vi "Test OOP API.vi"() -> ()   [LabVIEW 2019, in "Panther Dashboard.lvlib"]
uses:
  Panther Dashboard.lvlib
  <vilib>/National Instruments/Tree Map/API/List Roots.vi
  <vilib>/National Instruments/Tree Map/Utility/Into Tree Control Items.vi
  Class/VI/VI.lvclass
  Class/Library/Library.lvclass
  Class/Project/Project.lvclass
  <vilib>/National Instruments/Tree Map/Tree Map.lvlib
panel:
  in  "Modules Tree":string(tree)
  in  "error in":errorcluster
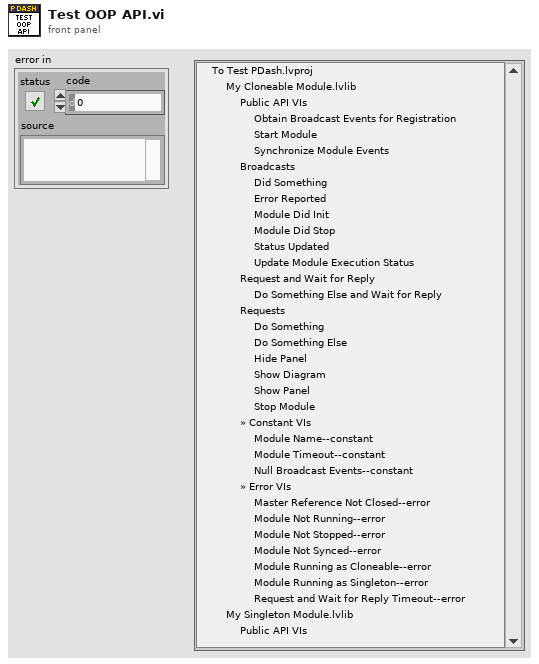
[diagram p1: front panel]
types:
  T1 = typedef "DQMH_Scripting API.lvlib/Module Information--cluster.ctl" = cluster{"Library":refnum<vi>, "Qualified Name":string, "Path":path, "Cloneable":bool, "Under Dependencies":bool}
  T2 = typedef "Tree Map.lvlib/Tree Map Data.ctl" = map{string, cluster{"Child Paths Set":set{string}, "Name":string, "Data":string, "Attributes":map{string, string}}}
  T3 = cluster{"Left Cell String":string, "Child Text":string[], "Child Tag":string, "Item Indent":i32, "Child Only?":bool, "Glyph Index":i32}[]
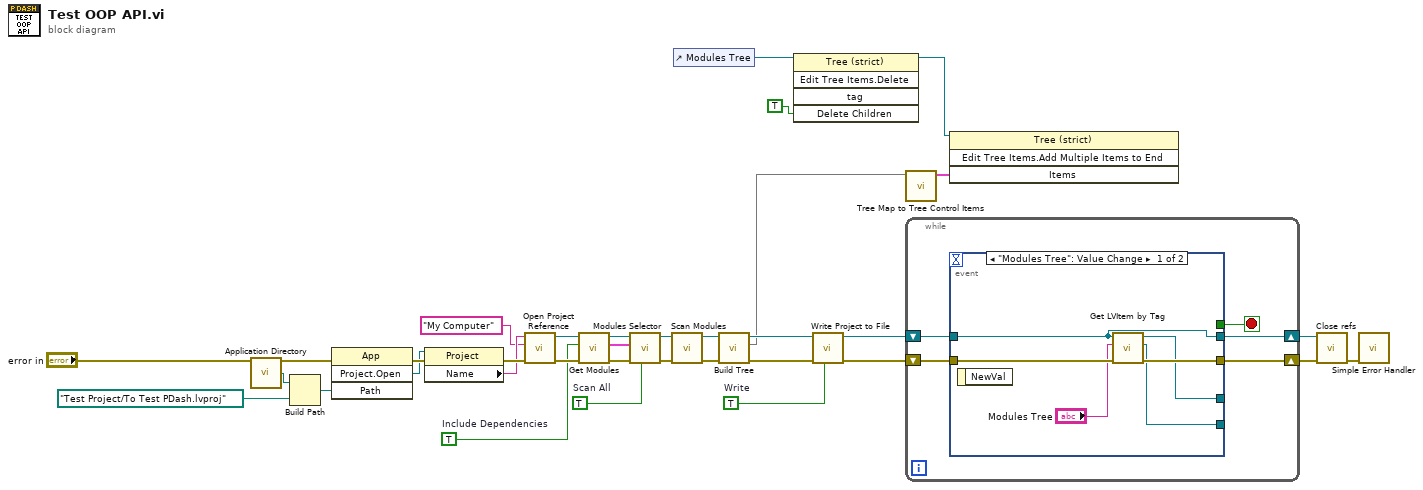
[diagram p0: block diagram]
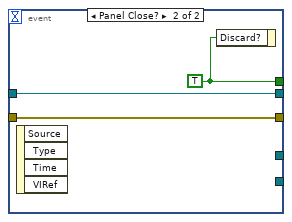
[diagram p2: hidden frame]
diagram:
  w2 = TRUE  # Write
  w19 = TRUE  # Scan All
  w17 = TRUE  # Include Dependencies
  n1 = call <vilib>:"Application Directory.vi"() -> ("Application Directory"=w16:path)
  n2 = Build Path(base path=w16, name or relative path=path "Test Project/To Test PDash.lvproj") -> (appended path=w14:path)
  n3 = invoke class="App" method="Project.Open"(error in="error in", "Path"=w14) -> (error out=w32:errorcluster, "Project:Open"=w13:refnum<vi>)  [unwired: 2 in, 2 out]
  n4 = property class="Project"(reference=w13, error in=w32) -> (error out=w30:errorcluster, "Name"=w12:string)  [unwired: 1 out]
  n5 = call "Open Project Reference.vi"("error in"=w30, "Target Selection"="My Computer", "Project Selection"=w12) -> ("error out"=w33:errorcluster, "Project"=w22:refnum<class "Project.lvclass">)  [unwired: 7 in]
  n6 = call "Get Modules.vi"("error in"=w33, "Include Dependencies"=w17, "Project in"=w22) -> ("error out"=w28:errorcluster, "DQMH Modules"=w20:T1[], "Project out"=w21:refnum<class "Project.lvclass">)  [unwired: 6 in]
  n7 = call "Modules Selector.vi"("Scan All"=w19, "error in"=w28, "DQMH Modules"=w20, "Project In"=w21) -> ("error out"=w27:errorcluster, "Project Out"=w18:refnum<class "Project.lvclass">)  [unwired: 5 in, 1 out]
  n8 = call "Scan Modules.vi"("error in (no error)"=w27, "Project In"=w18) -> ("error out"=w26:errorcluster, "Project Out"=w10:refnum<class "Project.lvclass">)  [unwired: 8 in]
  n9 = control-ref of="Modules Tree"() -> (w8:refnum<vi>)
  n10 = call "Build Tree.vi"("error in"=w26, "Project in"=w10) -> ("error out"=w24:errorcluster, "Tree Map Out"=w1:T2, "Project Out"=w4:refnum<class "Project.lvclass">)  [unwired: 7 in]
  n11 = invoke class="Tree (strict)" method="Edit Tree Items.Delete"(reference=w8, "Delete Children"=TRUE ("Delete Children?")) -> (reference out=w7:refnum<vi>)  [unwired: 3 in, 4 out]
  n12 = call "Write Project to File.vi"("Write"=w2, "error in"=w24, "Project In"=w4) -> ("error out"=w23:errorcluster, "Project Out"=w3:refnum<class "Project.lvclass">)  [unwired: 6 in, 1 out]
  n13 = call <vilib>:"Tree Map to Tree Control Items.vi"("Tree Map In"=w1) -> ("Tree Control Items"=w9:T3)  [unwired: 10 in]
  n14 = while {
    shift-right: [w37] -> w25
    shift-left: w23 -> [w38]
    shift-right: [w34] -> w5
    shift-left: w3 -> [w35]
    stop <- w36 stop-if-true
    n15 = event shown="[0] \"Modules Tree\": Value Change" {
      selector: _ -> [_ _]
      dyn-events: _ -> [_ _]
      timeout: _ -> [_ _]
      tunnel: w38 -> [w44 w47]
      tunnel: [w43 w47] -> w37
      tunnel: [_ w46] -> w36
      tunnel: w35 -> [w40 w45]
      tunnel: [w40 w45] -> w34
      tunnel: [w41 _] -> _
      tunnel: [w39 _] -> _
      event "Modules Tree": Value Change {
        n16 = event-data() -> ()  [unwired: 1 in, 1 out]
        n17 = call "Get LVItem by Tag.vi"("error in"=w44, "Tag"="Modules Tree", "Project in"=w40) -> ("error out"=w43:errorcluster, "Selected Library"=w41:refnum<class "Library.lvclass">, "Selected VI"=w39:refnum<class "VI.lvclass">)  [unwired: 6 in]
      }
      event Panel Close? {
        w46 = TRUE ("Discard?")
        n18 = event-data() -> ()  [unwired: 1 in, 4 out]
        n19 = event-data("Discard?"=w46) -> ()  [unwired: 1 in, 1 out]
      }
    }
  }
  n20 = invoke on="Invoke Node" class="Tree (strict)" method="Edit Tree Items.Add Multiple Items to End"(reference=w7, "Items"=w9) -> ()  [unwired: 2 in, 4 out]
  n21 = call "Close refs.vi"("error in"=w25, "Project"=w5) -> ("error out"=w29:errorcluster)  [unwired: 9 in]
  n22 = call <vilib>:"Simple Error Handler.vi"("error in (no error)"=w29) -> ()  [unwired: 4 in, 5 out]
